vi "Load Known Packages.vi"(8 "error in (no error)":errorcluster) -> (0 "error out":errorcluster, 1 "Success?":bool, 3 "Package Array from File":T1[](array[typedef]))   [LabVIEW 2019]
doc: "Load package info from file."
uses:
  Ctl/Ctl_Package Identifier Cluster.ctl
  <vilib>/Utility/file.llb/Read Delimited Spreadsheet (string).vi
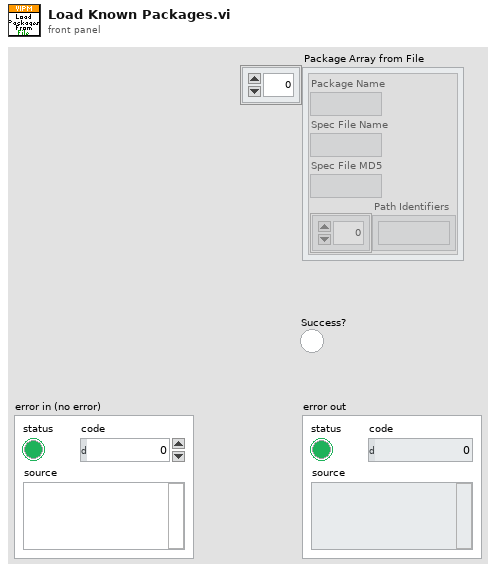
[diagram p1: front panel]
types:
  T1 = typedef "Ctl_Package Identifier Cluster.ctl" = cluster{"Package Name":string, "Spec File Name":string, "Spec File MD5":string, "Path Identifiers":string[]}
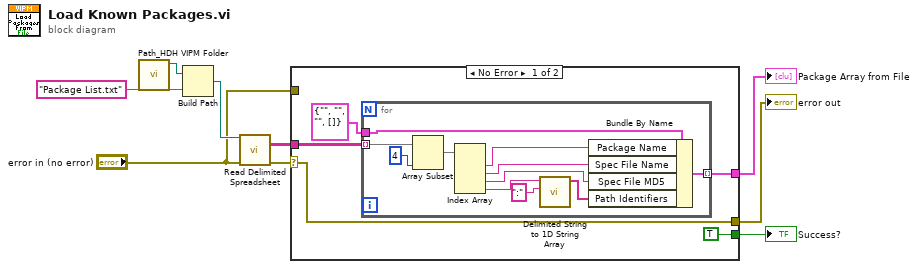
[diagram p0: block diagram]
diagram:
  n1 = call "Path_HDH VIPM Folder.vi"() -> ("HDH\\VIPM path"=w6:path)  [unwired: 10 in, 1 out]
  n2 = Build Path(base path=w6, name or relative path="Package List.txt") -> (appended path=w8:path)
  n3 = call-poly <vilib>:"Read Delimited Spreadsheet.vi"("file path (dialog if empty)"=w8, "error in (no error)"="error in (no error)") -> ("all rows"=w9:string[][], "error out"=w5:errorcluster)  [unwired: 8 in, 4 out]
  n4 = case shown="No Error" w5 {
    selector: w5 -> [w11 _]
    tunnel: [w14 _] -> w2
    tunnel: w9 -> [w12 _]
    tunnel: [w11 w26] -> w4
    tunnel: "error in (no error)" -> [_ w26]
    tunnel: [TRUE _] -> w1
    frame No Error {
      n5 = for {
        tunnel: w12 -> [w25] mode=indexing
        tunnel: T1 {"Package Name"="", "Spec File Name"="", "Spec File MD5"="", "Path Identifiers"=[]} -> [w20]
        tunnel: [w16] -> w14 mode=indexing
        n6 = Array Subset(array=w25, length=4) -> (w23:string[])  [unwired: 1 in]
        n7 = Index Array(array=w23) -> (element #1=w19:string, element #2=w15:string, element #3=w18:string, element #4=w22:string)  [unwired: 4 in]
        n8 = call <vilib>:"Delimited String to 1D String Array.vi"("delimiter"=":", "delimited string"=w22) -> ("string array"=w17:string[])  [unwired: 9 in]
        n9 = Bundle By Name(cluster=w20, "Package Name"=w19, "Spec File Name"=w15, "Spec File MD5"=w18, "Path Identifiers"=w17) -> (w16:T1)
      }
    }
    frame Error {
    }
  }
  "error out" <- w4
  "Package Array from File" <- w2
  "Success?" <- w1
